vi "ProStaMa_201130.vi"() -> ()   [LabVIEW 2017]
panel:
  in  "ON/OFF Current":bool
  in  "Stop program":bool
  in  "Current (A)":dbl
  in  "VISA name":refnum<visa-resource-name>="TCPIP0::192.168.0.104::inst0::INSTR"
  # "N5745A Power Supply"
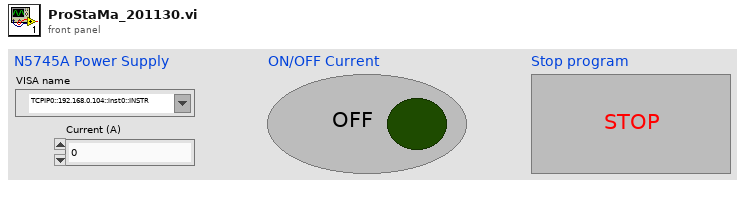
[diagram p1: front panel]
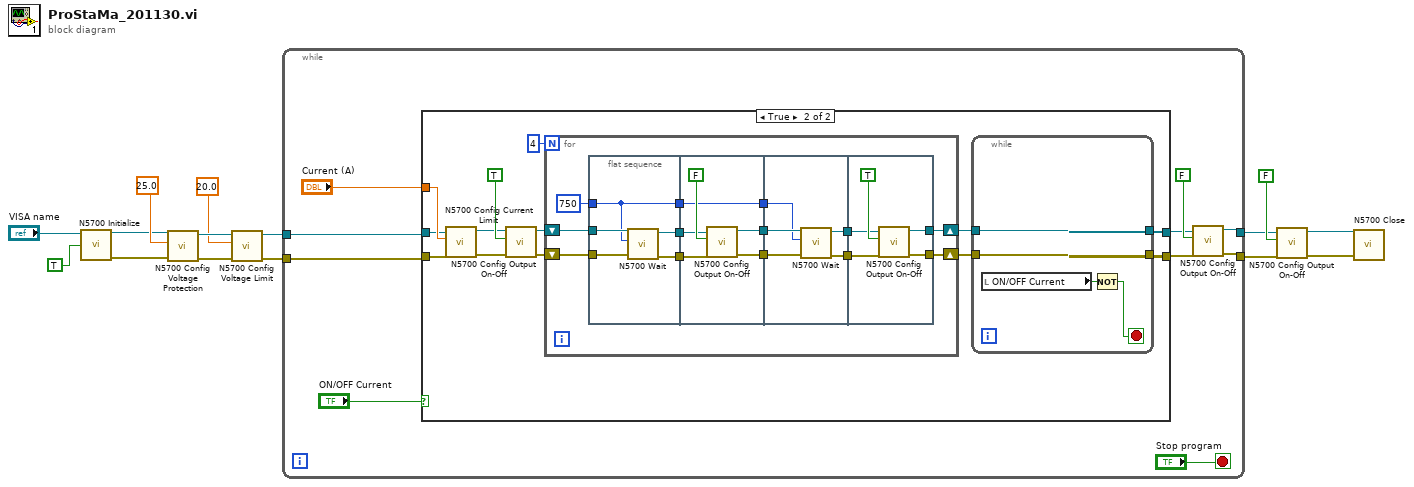
[diagram p0: block diagram]
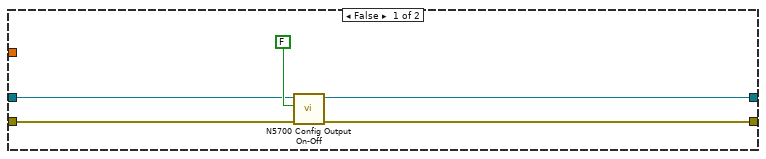
[diagram p2: hidden frame]
diagram:
  n1 = call <instrlib>:"N5700 Initialize.vi"("VISA name"="VISA name", "Reset (T)"=TRUE) -> ("VISA out"=w7:refnum<visa-resource-name>, "error out"=w6:errorcluster)  [unwired: 12 in]
  n2 = call <instrlib>:"N5700 Config Voltage Protection.vi"("error"=w6, "OVP Level"=25.0, "VISA"=w7) -> ("error out"=w13:errorcluster, "VISA out"=w12:refnum<visa-resource-name>)  [unwired: 4 in]
  n3 = call <instrlib>:"N5700 Config Voltage Limit.vi"("error"=w13, "Volt Limit"=20.0 ("Voltage Limit"), "VISA"=w12) -> ("error out"=w9:errorcluster, "VISA out"=w8:refnum<visa-resource-name>)  [unwired: 4 in]
  n4 = while {
    tunnel: w9 -> [w23]
    tunnel: w8 -> [w24]
    tunnel: [w17] -> w4
    tunnel: [w16] -> w2
    stop <- "Stop program" stop-if-true
    n5 = case shown="True" "ON/OFF Current" {
      tunnel: "Current (A)" -> [_ w43]
      tunnel: w23 -> [w26 w42]
      tunnel: w24 -> [w29 w41]
      tunnel: [w28 w33] -> w19
      tunnel: [w27 w31] -> w18
      frame False {
        n6 = call <instrlib>:"N5700 Config Output On-Off.vi"("error"=w26, "Output ON"=FALSE, "VISA"=w29) -> ("error out"=w27:errorcluster, "VISA out"=w28:refnum<visa-resource-name>)  [unwired: 4 in]
      }
      frame True {
        n7 = call <instrlib>:"N5700 Config Current Limit.vi"("error"=w42, "Current Limit"=w43, "VISA"=w41) -> ("error out"=w37:errorcluster, "VISA out"=w39:refnum<visa-resource-name>)  [unwired: 4 in]
        n8 = call <instrlib>:"N5700 Config Output On-Off.vi"("error"=w37, "Output ON"=TRUE, "VISA"=w39) -> ("error out"=w36:errorcluster, "VISA out"=w38:refnum<visa-resource-name>)  [unwired: 4 in]
        n9 = for {
          N: 4 -> [_]
          shift-right: [w52] -> w34
          shift-left: w38 -> [w54]
          shift-right: [w51] -> w32
          shift-left: w36 -> [w53]
          n10 = flat-sequence {
            tunnel: [w65] -> w60
            tunnel: [w64] -> w59
            tunnel: w54 -> [w63]
            tunnel: w53 -> [w62]
            tunnel: u32 750 ("Delay (20 mS)") -> [w61]
            tunnel: [w61] -> w48
            tunnel: w60 -> [w70]
            tunnel: w59 -> [w69]
            tunnel: [w68] -> w58
            tunnel: [w67] -> w57
            tunnel: [w66] -> w49
            tunnel: w48 -> [w66]
            tunnel: w58 -> [w76]
            tunnel: w57 -> [w75]
            tunnel: [w74] -> w56
            tunnel: [w73] -> w55
            tunnel: w49 -> [w72]
            tunnel: w56 -> [w79]
            tunnel: w55 -> [w80]
            tunnel: [w78] -> w52
            tunnel: [w77] -> w51
            frame #0 {
              n11 = call <instrlib>:"N5700 Wait.vi"("error"=w62, "Delay (20 mS)"=w61, "VISA"=w63) -> ("error out"=w64:errorcluster, "VISA out"=w65:refnum<visa-resource-name>)  [unwired: 4 in]
            }
            frame #1 {
              n12 = call <instrlib>:"N5700 Config Output On-Off.vi"("error"=w69, "Output ON"=FALSE, "VISA"=w70) -> ("error out"=w67:errorcluster, "VISA out"=w68:refnum<visa-resource-name>)  [unwired: 4 in]
            }
            frame #2 {
              n13 = call <instrlib>:"N5700 Wait.vi"("error"=w75, "Delay (20 mS)"=w72, "VISA"=w76) -> ("error out"=w74:errorcluster, "VISA out"=w73:refnum<visa-resource-name>)  [unwired: 4 in]
            }
            frame #3 {
              n14 = call <instrlib>:"N5700 Config Output On-Off.vi"("error"=w79, "Output ON"=TRUE, "VISA"=w80) -> ("error out"=w77:errorcluster, "VISA out"=w78:refnum<visa-resource-name>)  [unwired: 4 in]
            }
          }
        }
        n15 = while {
          tunnel: w34 -> [w47]
          tunnel: [w47] -> w33
          tunnel: w32 -> [w46]
          tunnel: [w46] -> w31
          stop <- w44 stop-if-true
          n16 = local read "ON/OFF Current"() -> (w45:bool)
          n17 = Not(x=w45) -> (.not. x?=w44:bool)
        }
      }
    }
    n18 = call <instrlib>:"N5700 Config Output On-Off.vi"("error"=w18, "Output ON"=FALSE, "VISA"=w19) -> ("error out"=w16:errorcluster, "VISA out"=w17:refnum<visa-resource-name>)  [unwired: 4 in]
  }
  n19 = call <instrlib>:"N5700 Config Output On-Off.vi"("error"=w2, "Output ON"=FALSE, "VISA"=w4) -> ("error out"=w1:errorcluster, "VISA out"=w3:refnum<visa-resource-name>)  [unwired: 4 in]
  n20 = call <instrlib>:"N5700 Close.vi"("error"=w1, "VISA name"=w3) -> ()  [unwired: 6 in, 1 out]
